vi "Far Right Rocket.vi"() -> (4 "path":cluster{"X":dbl, "Y":dbl}[](array[cluster])=[{"X"=68.0, "Y"=162.0}, {"X"=68.99922222003843, "Y"=161.96074883622666}, {"X"=69.9984371509684, "Y"=161.92149577286008}, {"X"=70.99765336101497, "Y"=161.88223940219427}, {"X"=71.99687771262886, "Y"=161.84297995456467}, {"X"=72.99611219846692, "Y"=161.80371888599015}, {"X"=73.99535367467291, "Y"=161.76445802412644}, {"X"=74.99459606588916, "Y"=161.72519874216525}, {"X"=75.99383356469386, "Y"=161.6859415033598}, {"X"=76.99306320652555, "Y"=161.64668587954515}, {"X"=77.99228580323073, "Y"=161.6074309264887}, {"X"=78.99150512235313, "Y"=161.56817568234683}, {"X"=79.99072595349125, "Y"=161.52891956181264}, {"X"=80.98995203445003, "Y"=161.4896625128224}, {"X"=81.98918468425585, "Y"=161.45040492568972}, {"X"=82.98842256048138, "Y"=161.41114738220054}, {"X"=83.98766245649233, "Y"=161.37189037430284}, {"X"=84.98690068315092, "Y"=161.33263410655596}, {"X"=85.98613444630836, "Y"=161.29337844267886}, {"X"=86.98536274808941, "Y"=161.25412300143486}, {"X"=87.98458624501566, "Y"=161.2148671418304}, {"X"=88.98380953629679, "Y"=161.1756119249571}, {"X"=89.98302462726822, "Y"=161.1363501367438}, {"X"=90.98226773320192, "Y"=161.09710459198016}, {"X"=91.98147096303573, "Y"=161.0578277010583}, {"X"=92.98072221068904, "Y"=161.0185839657486}, {"X"=93.97996452789548, "Y"=160.979329458069}, {"X"=94.97918668205918, "Y"=160.9400618174647}, {"X"=95.97841843829598, "Y"=160.90080521333388}, {"X"=96.97766086945505, "Y"=160.86155812676282}, {"X"=97.97689449735313, "Y"=160.82230545752435}, {"X"=98.9761131412384, "Y"=160.78304407488093}, {"X"=99.9753286064865, "Y"=160.7437828178918}, {"X"=100.97454830879028, "Y"=160.70452469846595}, {"X"=101.97378169980823, "Y"=160.66527485137823}, {"X"=102.97300839357722, "Y"=160.6260119355682}, {"X"=103.9722276124876, "Y"=160.58675184769797}, {"X"=104.9714670279113, "Y"=160.54748832513013}, {"X"=105.97068237877795, "Y"=160.5082193373712}, {"X"=106.96989848276343, "Y"=160.468955469187}, {"X"=107.96913664321573, "Y"=160.42969662129994}, {"X"=108.96837099340783, "Y"=160.39043399520145}, {"X"=109.96758137204623, "Y"=160.35116384088028}, {"X"=110.96677953266466, "Y"=160.31188841925157}, {"X"=111.96598213691128, "Y"=160.27260962131297}, {"X"=112.96518773790544, "Y"=160.23332667412228}, {"X"=113.96438416789229, "Y"=160.19403769264756}, {"X"=114.96356533414324, "Y"=160.15474048029617}, {"X"=115.96273481570643, "Y"=160.11543196958047}, {"X"=116.96189695284873, "Y"=160.07610819112173}, {"X"=117.9610486679224, "Y"=160.0367651418005}, {"X"=118.96017974457399, "Y"=159.99739921967532}, {"X"=119.9592787432485, "Y"=159.95800637692184}, {"X"=120.95833759561192, "Y"=159.91858060937255}, {"X"=121.95735111190099, "Y"=159.8791129294992}, {"X"=122.95631275297609, "Y"=159.83959124999987}, {"X"=123.95521040390531, "Y"=159.80000065133308}, {"X"=124.95402475032796, "Y"=159.76032322149203}, {"X"=125.9527302103382, "Y"=159.72053707363634}, {"X"=126.95129650827181, "Y"=159.68061471534864}, {"X"=127.9496888554509, "Y"=159.6405211738704}, {"X"=128.9478658524024, "Y"=159.60021209772344}, {"X"=129.94577555172773, "Y"=159.55963170050524}, {"X"=130.9433507726822, "Y"=159.51871016769758}, {"X"=131.94050453954597, "Y"=159.47736012612415}, {"X"=132.9371257709694, "Y"=159.43547190729686}, {"X"=133.93307459888345, "Y"=159.3929074689073}, {"X"=134.92817630720361, "Y"=159.34949285707637}, {"X"=135.9222129163882, "Y"=159.30500896925398}, {"X"=136.9149117212169, "Y"=159.2591801623536}, {"X"=137.90593035395466, "Y"=159.2116600154721}, {"X"=138.89483799774644, "Y"=159.16201335085697}, {"X"=139.8810921567236, "Y"=159.10969344489988}, {"X"=140.86400996097825, "Y"=159.05401318702985}, {"X"=141.84273245888713, "Y"=158.99410871330224}, {"X"=142.81617981732063, "Y"=158.92889370077378}, {"X"=143.78299483800822, "Y"=158.85700202188804}, {"X"=144.74147166191685, "Y"=158.77671580564228}, {"X"=145.68946588358668, "Y"=158.68587512319436}, {"X"=146.62428143202294, "Y"=158.5817644938013}, {"X"=147.54252840425667, "Y"=158.46097015916794}, {"X"=148.4399444918261, "Y"=158.31920054140917}, {"X"=149.3111706594316, "Y"=158.15106039414965}, {"X"=150.1494692502334, "Y"=157.94976676183217}, {"X"=150.94636960551003, "Y"=157.70679183601874}, {"X"=151.69122245292547, "Y"=157.4114139680779}, {"X"=152.3706395355201, "Y"=157.05015326002385}, {"X"=152.96778895703363, "Y"=156.60606205939004}, {"X"=153.49975928271206, "Y"=156.05633029687527}, {"X"=153.9798868795653, "Y"=155.4225722587485}, {"X"=154.41877942636353, "Y"=154.72197981303913}, {"X"=154.82487409654715, "Y"=153.96822734145724}, {"X"=155.20488158933327, "Y"=153.17219149508284}, {"X"=155.56413937634372, "Y"=152.34252364675427}, {"X"=155.9068927283217, "Y"=151.48610517770464}, {"X"=156.2365182730088, "Y"=150.60840958144848}, {"X"=156.55570181199874, "Y"=149.71379046760447}, {"X"=156.86657972949084, "Y"=148.80571064458076}, {"X"=157.17085142780758, "Y"=147.88692434988562}, {"X"=157.46986871722802, "Y"=146.95962222013912}, {"X"=157.76470688689326, "Y"=146.02554662267235}, {"X"=158.05622122347262, "Y"=145.0860834054644}, {"X"=158.34509197452365, "Y"=144.14233488039767}, {"X"=158.63186013576242, "Y"=143.195177870337}, {"X"=158.91695594670927, "Y"=142.24530986988307}, {"X"=159.20072158483828, "Y"=141.29328574982142}, {"X"=159.48342923631878, "Y"=140.33954694206253}, {"X"=159.7652954765285, "Y"=139.38444464836437}, {"X"=160.0464927025721, "Y"=138.42825830151352}, {"X"=160.32715821159314, "Y"=137.47121025587592}, {"X"=160.60740140278767, "Y"=136.51347748293605}, {"X"=160.88730948949464, "Y"=135.55520088698913}, {"X"=161.16695203406184, "Y"=134.59649272879813}, {"X"=161.44638455765318, "Y"=133.6374425444746}, {"X"=161.7256514266072, "Y"=132.6781218677792}, {"X"=162.00478817452148, "Y"=131.7185880020338}, {"X"=162.28382338394653, "Y"=130.7588870391752}, {"X"=162.5627802229444, "Y"=129.79905628515957}, {"X"=162.8416777094818, "Y"=128.83912622059714}, {"X"=163.12053176024423, "Y"=127.8791221014003}, {"X"=163.39935606933963, "Y"=126.919065285116}, {"X"=163.67816285557956, "Y"=125.95897435364704}, {"X"=163.956963513806, "Y"=124.99886609161393}, {"X"=164.235769203667, "Y"=124.03875637167809}, {"X"=164.5145914135225, "Y"=123.07866099143854}, {"X"=164.79344252495275, "Y"=122.11859650962067}, {"X"=165.07233644100236, "Y"=121.15858111052677}, {"X"=165.35128926328434, "Y"=120.19863557833975}, {"X"=165.6303201485933, "Y"=119.23878435800164}, {"X"=165.90945227993004, "Y"=118.27905688023421}, {"X"=166.1887141030744, "Y"=117.31948907060281}, {"X"=166.46814084488605, "Y"=116.36012525379934}, {"X"=166.74777637681646, "Y"=115.40102049438406}, {"X"=167.02767555010558, "Y"=114.44224347911593}, {"X"=167.3079071123382, "Y"=113.48388013574193}, {"X"=167.5885573393311, "Y"=112.52603816780783}, {"X"=167.86973458029243, "Y"=111.56885272223657}, {"X"=168.15157496377094, "Y"=110.61249349845977}, {"X"=168.43424955983684, "Y"=109.6571736845921}, {"X"=168.7179733713687, "Y"=108.70316118338991}, {"X"=169.00301663320167, "Y"=107.75079271056005}, {"X"=169.28971902130024, "Y"=106.80049151112352}, {"X"=169.5785075215324, "Y"=105.85278963293156}, {"X"=169.8699188965236, "Y"=104.9083559295638}, {"X"=170.16462793260882, "Y"=103.96803126239266}, {"X"=170.4634829552912, "Y"=103.03287275345467}, {"X"=170.76755048327607, "Y"=102.10420942101224}, {"X"=171.0781713694406, "Y"=101.18371212847494}, {"X"=171.39703138036296, "Y"=100.27348152761628}, {"X"=171.72624992695955, "Y"=99.3761586223287}, {"X"=172.06849161589625, "Y"=98.49506377065862}, {"X"=172.42710649342874, "Y"=97.63437144143442}, {"X"=172.80630636323298, "Y"=96.79932992421135}, {"X"=173.21138645802048, "Y"=95.99653755638406}, {"X"=173.64900413197097, "Y"=95.23429000491143}, {"X"=174.12752924279224, "Y"=94.52301687976738}, {"X"=174.65748466588826, "Y"=93.87583065871118}, {"X"=175.25210012681814, "Y"=93.30921681493415}, {"X"=175.92889342498262, "Y"=92.84085079829725}, {"X"=176.67105061587696, "Y"=92.45063068897755}, {"X"=177.46519795414542, "Y"=92.12256750511004}, {"X"=178.30069801552273, "Y"=91.84394367704446}, {"X"=179.16908983592845, "Y"=91.60464370152425}, {"X"=180.06364360094324, "Y"=91.39662174715677}, {"X"=180.97900644786094, "Y"=91.21347819060406}, {"X"=181.91092073787985, "Y"=91.05012279596038}, {"X"=182.85599997027984, "Y"=90.9025068096627}, {"X"=183.8115505444419, "Y"=90.76740987021854}, {"X"=184.77542998893537, "Y"=90.64227051703541}, {"X"=185.7459341965071, "Y"=90.52505137752124}, {"X"=186.72170773059153, "Y"=90.41413193703855}, {"X"=187.70167248323548, "Y"=90.30822324819607}, {"X"=188.68497093004356, "Y"=90.2063000906923}, {"X"=189.67092099582126, "Y"=90.10754701132487}, {"X"=190.65898015549797, "Y"=90.01131540423965}, {"X"=191.64871688085657, "Y"=89.91708937254064}, {"X"=192.6397879301201, "Y"=89.82445857458879}, {"X"=193.63192028490084, "Y"=89.73309662599044}, {"X"=194.6248967835455, "Y"=89.64274392070188}, {"X"=195.61854469439896, "Y"=89.55319396722814}, {"X"=196.61272662722874, "Y"=89.4642825208129}, {"X"=197.60733330413342, "Y"=89.37587893956946}, {"X"=198.60227780922443, "Y"=89.28787930947284}, {"X"=199.59749101432766, "Y"=89.20020097619661}, {"X"=200.5929179399902, "Y"=89.11277819584497}, {"X"=201.58851486043042, "Y"=89.02555867556163}, {"X"=202.58424700030088, "Y"=88.93850082189192}, {"X"=203.5800867023161, "Y"=88.8515715520586}, {"X"=204.57601196956338, "Y"=88.76474455295948}, {"X"=205.57200530599175, "Y"=88.67799889626059}, {"X"=206.56805279421604, "Y"=88.59131793670556}, {"X"=207.56414336218853, "Y"=88.50468843567333}, {"X"=208.56026820021478, "Y"=88.41809986390842}, {"X"=209.55642029743203, "Y"=88.33154384666696}, {"X"=210.55259407417148, "Y"=88.2450137228035}, {"X"=211.548785087284, "Y"=88.15850419189866}, {"X"=212.54498980366307, "Y"=88.07201104025515}, {"X"=213.54120540210198, "Y"=87.9855309062545}, {"X"=214.53742964997898, "Y"=87.89906112672182}, {"X"=215.5336607551778, "Y"=87.81259956473144}, {"X"=216.52989730104102, "Y"=87.72614452784961}, {"X"=217.5261381598811, "Y"=87.63969466507999}, {"X"=218.52238242663938, "Y"=87.5532488896764}, {"X"=219.51862938319547, "Y"=87.46680633574816}, {"X"=220.51487845815768, "Y"=87.38036631017572}, {"X"=221.51112918838834, "Y"=87.29392824817369}, {"X"=222.50738119680204, "Y"=87.20749168752656}, {"X"=223.50363417670658, "Y"=87.1210562495836}, {"X"=224.499887872804, "Y"=87.03462161647113}, {"X"=225.49614206353843, "Y"=86.94818751024842}, {"X"=226.49239655019974, "Y"=86.86175367962042}, {"X"=227.4886511494427, "Y"=86.77531988994818}, {"X"=228.4849056839532, "Y"=86.68888591070234}, {"X"=229.4811599711814, "Y"=86.6024515005907}, {"X"=230.47741381303837, "Y"=86.51601639363655}, {"X"=231.47366698711323, "Y"=86.42958028657158}, {"X"=232.46991923693437, "Y"=86.34314282451017}, {"X"=233.46617025883845, "Y"=86.25670358211944}, {"X"=234.46241968508195, "Y"=86.17026203985648}, {"X"=235.45866706387318, "Y"=86.08381755585853}, {"X"=236.45491183603767, "Y"=85.99736933278471}, {"X"=237.45115330645325, "Y"=85.91091637701554}, {"X"=238.44739060770434, "Y"=85.82445744683803}, {"X"=239.4436226537558, "Y"=85.7379909865852}, {"X"=240.43984808180065, "Y"=85.65151504395355}, {"X"=241.43606517997142, "Y"=85.56502716695766}, {"X"=242.43227179732398, "Y"=85.47852427526512}, {"X"=243.42846523099473, "Y"=85.39200249865941}, {"X"=244.4246420841032, "Y"=85.30545697356102}, {"X"=245.42079808676397, "Y"=85.21888158674717}, {"X"=246.41692787101624, "Y"=85.13226865308671}, {"X"=247.4130246881821, "Y"=85.04560851075753}, {"X"=248.40908005393152, "Y"=84.95888901282878}, {"X"=249.40508330224165, "Y"=84.87209488830123}, {"X"=250.40102102449475, "Y"=84.78520693867115}, {"X"=251.39687636397903, "Y"=84.69820102752249}, {"X"=252.39262812865204, "Y"=84.61104680998783}, {"X"=253.38824967560973, "Y"=84.52370613540288}, {"X"=254.38370750872156, "Y"=84.43613103927795}, {"X"=255.3789595156857, "Y"=84.3482612189688}, {"X"=256.37395275166773, "Y"=84.26002086009626}, {"X"=257.36862065274204, "Y"=84.17131464652512}, {"X"=258.3628795323976, "Y"=84.08202274378223}, {"X"=259.356624176714, "Y"=83.99199449187529}, {"X"=260.34972230646275, "Y"=83.90104047563987}, {"X"=261.34200761478104, "Y"=83.80892255537981}, {"X"=262.33327101405143, "Y"=83.71534133316665}, {"X"=263.3232496313066, "Y"=83.61992039512444}, {"X"=264.3116129729172, "Y"=83.52218650027872}, {"X"=265.2979455303196, "Y"=83.42154467320287}, {"X"=266.2817249112521, "Y"=83.31724688950537}, {"X"=267.2622943455009, "Y"=83.2083527060375}, {"X"=268.23882811812194, "Y"=83.09367976377865}, {"X"=269.2102881108665, "Y"=82.97174155834328}, {"X"=270.17536916453145, "Y"=82.84066920290599}, {"X"=271.13243038655304, "Y"=82.69811306579825}, {"X"=272.07940878841686, "Y"=82.54111910577039}, {"X"=273.01371070743613, "Y"=82.36597339620668}, {"X"=273.93207529823104, "Y"=82.16800665532637}, {"X"=274.83040290924396, "Y"=81.94134849448528}, {"X"=275.7035393114932, "Y"=81.6786184502986}, {"X"=276.54500442322353, "Y"=81.37053753914955}, {"X"=277.3466512528296, "Y"=81.00543988960987}, {"X"=278.1247631782456, "Y"=80.56635750688427}, {"X"=278.8841409083244, "Y"=80.06843096930913}, {"X"=279.628599141502, "Y"=79.52370379447778}, {"X"=280.36116733931806, "Y"=78.94175630862348}, {"X"=281.0842491716829, "Y"=78.33020987432378}, {"X"=281.7997490257473, "Y"=77.69512801482611}, {"X"=282.5091722367529, "Y"=77.04133554681422}, {"X"=283.21370431618493, "Y"=76.37267251809354}, {"X"=283.91427334714035, "Y"=75.69219631535154}, {"X"=284.61159883087356, "Y"=75.00234257924828}, {"X"=285.3062295553887, "Y"=74.3050533960501}, {"X"=285.99857247914133, "Y"=73.6018795127228}, {"X"=286.6889141500279, "Y"=72.89406195521428}, {"X"=287.3774357869619, "Y"=72.1825973456166}, {"X"=288.064222817793, "Y"=71.46829035595009}, {"X"=288.7492693755659, "Y"=70.75179605929992}, {"X"=289.43247798976404, "Y"=70.03365440731945}, {"X"=290.11365445629036, "Y"=69.31431864871621}, {"X"=290.79249761619775, "Y"=68.59417918443584}, {"X"=291.4685835051982, "Y"=67.87358411508204}, {"X"=292.1413430397279, "Y"=67.15285756201152}, {"X"=292.810032065139, "Y"=66.43231672636854}, {"X"=293.4736921896133, "Y"=65.71228858389443}, {"X"=294.1311003424216, "Y"=64.99312709418302}, {"X"=294.7807044017078, "Y"=64.27523183013155}, {"X"=295.4205415037918, "Y"=63.55906900808579}, {"X"=296.04813473448854, "Y"=62.84519602553392}, {"X"=296.6603627651486, "Y"=62.134290797810834}, {"X"=297.25329557217106, "Y"=61.427187437853696}, {"X"=297.82198759364275, "Y"=60.724920156890725}, {"X"=298.3602174366129, "Y"=60.02877769662455}, {"X"=298.86016043538456, "Y"=59.34037115775815}, {"X"=299.3119768270383, "Y"=58.66171879478159}, {"X"=299.7032938692021, "Y"=57.99535223990418}, {"X"=300.0185546432154, "Y"=57.34444974682944}, {"X"=300.238199268564, "Y"=56.71300346740602}, {"X"=300.33763543704265, "Y"=56.10602956423826}, {"X"=300.2859440763114, "Y"=55.529832221435704}, {"X"=300.070246518476, "Y"=54.96483272108132}, {"X"=299.72409924005257, "Y"=54.40873994447525}, {"X"=299.27419295811575, "Y"=53.8597315335168}, {"X"=298.7417573772689, "Y"=53.31635800763873}, {"X"=298.14367855852214, "Y"=52.777466448261706}, {"X"=297.49338766060686, "Y"=52.24213983000887}, {"X"=296.8015678328565, "Y"=51.709648763119084}, {"X"=296.076716490795, "Y"=51.17941309293592}, {"X"=295.3255925531682, "Y"=50.650971366805436}, {"X"=294.5535721703445, "Y"=50.12395655430162}, {"X"=293.76493167702665, "Y"=49.598076727225376}, {"X"=292.9630726653485, "Y"=49.07309969025507}, {"X"=292.15070101796135, "Y"=48.548840762062575}, {"X"=291.3299693211598, "Y"=48.025153058780255}, {"X"=290.50259015709435, "Y"=47.50191976244209}, {"X"=289.6699262403881, "Y"=46.97904796986119}, {"X"=288.8330621415436, "Y"=46.4564638027476}, {"X"=287.99286136974814, "Y"=45.93410852142105}, {"X"=287.1500118196141, "Y"=45.41193543432977}, {"X"=286.3050619754609, "Y"=44.88990743955875}, {"X"=285.45844977936366, "Y"=44.36799507069229}, {"X"=284.61052568157965, "Y"=43.84617494593402}, {"X"=283.76157108552235, "Y"=43.324428538583085}, {"X"=282.9118131579847, "Y"=42.80274120269961}, {"X"=282.06143678475456, "Y"=42.28110140192866}, {"X"=281.2105943014238, "Y"=41.759500101459544}, {"X"=280.35941351146835, "Y"=41.23793029209665}, {"X"=279.5080044131266, "Y"=40.716386621716005}, {"X"=278.6564649887819, "Y"=40.19486511422044}, {"X"=277.80488636163113, "Y"=39.67336296054686}, {"X"=276.9533575913549, "Y"=39.151878370540125}, {"X"=276.1019703614397, "Y"=38.63041047824247}, {"X"=275.25082380482877, "Y"=38.10895929607247}, {"X"=274.4000297216566, "Y"=37.58752571566293}, {"X"=273.54971846357677, "Y"=37.06611155506635}, {"X"=272.7000457940395, "Y"=36.54471965513018}, {"X"=271.8512010867312, "Y"=36.02335402729606}, {"X"=271.00341729149307, "Y"=35.50202006940595}, {"X"=270.15698319548386, "Y"=34.98072483779375}, {"X"=269.31225862564185, "Y"=34.459477440758796}, {"X"=268.46969337485575, "Y"=33.938289486070204}, {"X"=267.629850900368, "Y"=33.4171757256318}, {"X"=266.79343794735144, "Y"=32.89615481098364}, {"X"=265.9613417680151, "Y"=32.37525027554903}, {"X"=265.13467682019507, "Y"=31.854491784696148}, {"X"=264.31484340682033, "Y"=31.333916690228552}, {"X"=263.5036013839761, "Y"=30.813571991691234}, {"X"=262.70316279364374, "Y"=30.293516815573234}, {"X"=261.89958084807495, "Y"=29.763602722522062}, {"X"=261.09373833650307, "Y"=29.226037108805716}, {"X"=260.28639907103235, "Y"=28.68262465689814}, {"X"=259.47824809179536, "Y"=28.134862321084633}, {"X"=258.6699277180843, "Y"=27.584018116114073}, {"X"=257.862071350249, "Y"=27.031197853521927}, {"X"=257.0553368079468, "Y"=26.477403340570792}, {"X"=256.25044095621394, "Y"=25.923585107209753}, {"X"=255.44819743594, "Y"=25.370692435375645}, {"X"=254.6495594843195, "Y"=24.81972332180323}, {"X"=253.8556701030928, "Y"=24.27177700348432}])   [LabVIEW 2018]
uses:
  AutonBuilder/Typedef/Data Point.ctl
panel:
  in  "Data Points":T1[](array[typedef])=[{"X"=68.0, "Y"=162.0, "Theta"=0.0, "Speed %"=0.0, "Disabled?"=FALSE}, {"X"=154.20618556701032, "Y"=158.61324041811847, "Theta"=0.0, "Speed %"=0.0, "Disabled?"=FALSE}, {"X"=173.69072164948454, "Y"=91.44250871080139, "Theta"=0.0, "Speed %"=0.0, "Disabled?"=FALSE}, {"X"=277.7938144329897, "Y"=82.41114982578398, "Theta"=0.0, "Speed %"=0.0, "Disabled?"=FALSE}, {"X"=303.4020618556701, "Y"=55.31707317073171, "Theta"=0.0, "Speed %"=0.0, "Disabled?"=FALSE}, {"X"=262.7628865979382, "Y"=30.4808362369338, "Theta"=0.0, "Speed %"=0.0, "Disabled?"=FALSE}, {"X"=253.8556701030928, "Y"=24.27177700348432, "Theta"=0.0, "Speed %"=0.0, "Disabled?"=FALSE}]
  out "Graph":cluster{dbl[], dbl[]}[](graph)=[{[48.5, 82.0, 82.0, 48.5, 48.5], [176.25, 176.25, 147.75, 147.75, 176.25]}, {[68.0, 154.20618556701032, 173.69072164948454, 277.7938144329897, 303.4020618556701, 262.7628865979382, 253.8556701030928], [162.0, 158.61324041811847, 91.44250871080139, 82.41114982578398, 55.31707317073171, 30.4808362369338, 24.27177700348432]}, {array[360 elements], array[360 elements]}, {array[360 elements], array[360 elements]}, {array[360 elements], array[360 elements]}]
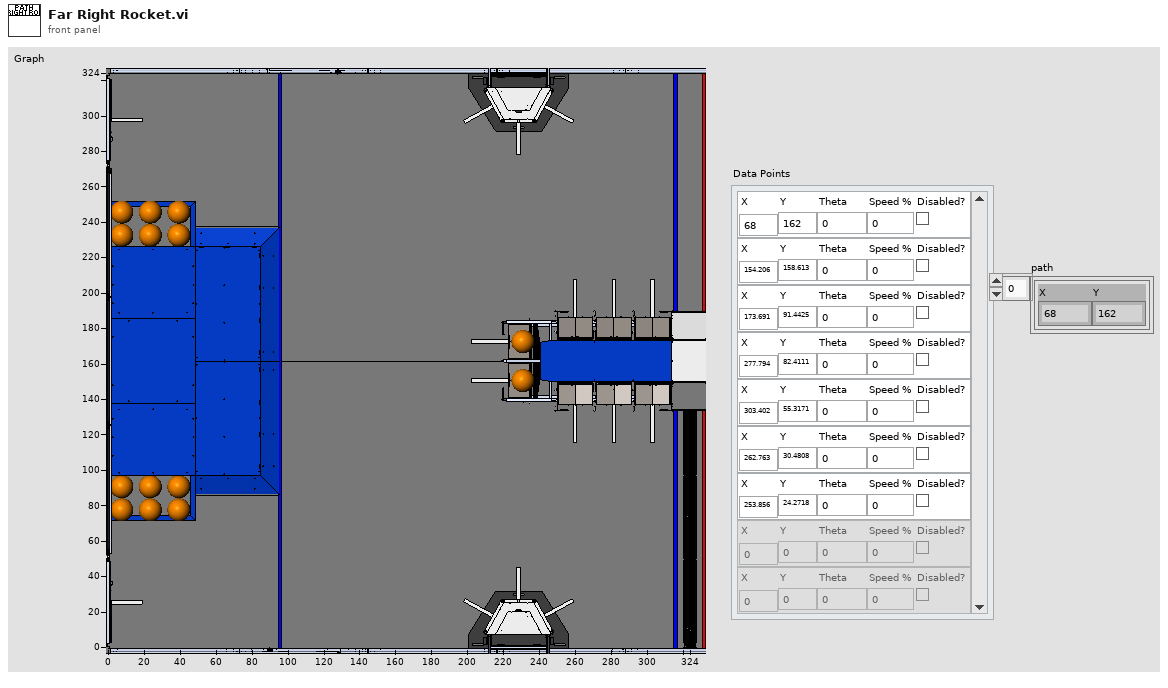
[diagram p1: front panel]
types:
  T1 = typedef "Data Point.ctl" = cluster{"X":dbl, "Y":dbl, "Theta":dbl, "Speed %":dbl, "Disabled?":bool}
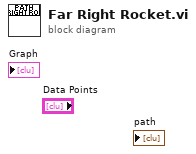
[diagram p0: block diagram]
diagram:
